vi "Supply_SetVolts.vi"(8 "error in (no error)":errorcluster, 9 "Command string":string, 10 "Volts IN [V]":dbl, 11 "KE2410 in":refnum<class "KE2410.lvclass">) -> (0 "error out":errorcluster, 2 "Compliance exceeded?":bool, 3 "KE2410 out":refnum<class "KE2410.lvclass">)   [LabVIEW 2018, in "KE2410.lvclass"]
uses:
  KE2410.lvclass
  InstrumentSetup.vi
  SupplyControl.lvclass
  InstrControl.lvclass
panel:
  out "Command sent":string
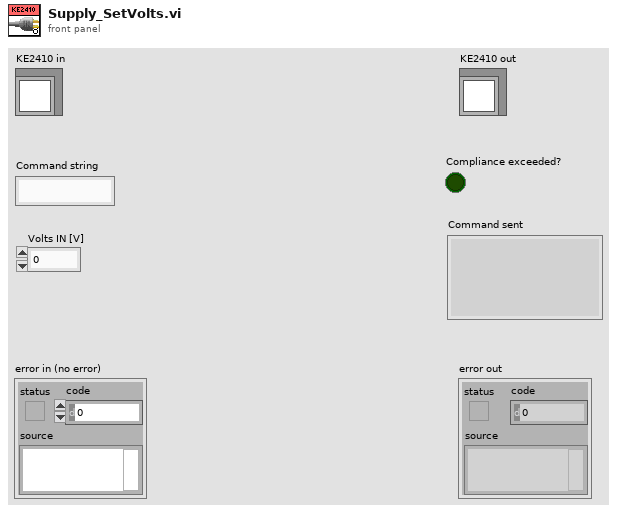
[diagram p1: front panel]
types:
  T1 = cluster{"Current Limit":sgl, "KE2410":refnum<class "KE2410.lvclass">}
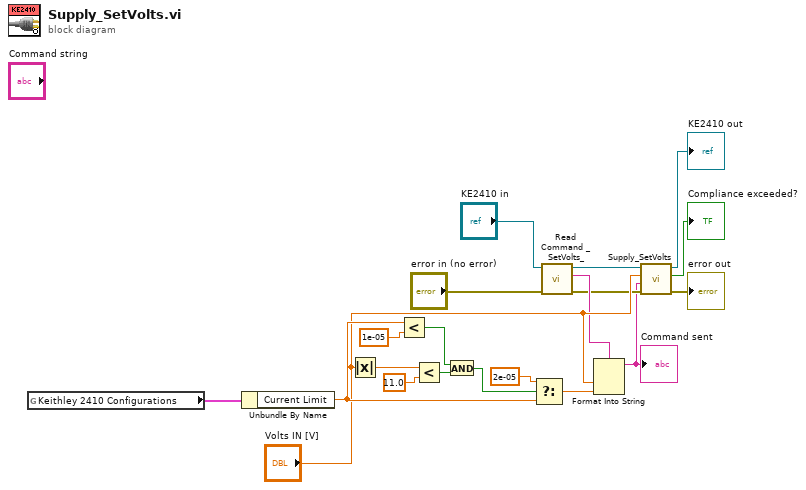
[diagram p0: block diagram]
diagram:
  n1 = global read "InstrumentSetup.vi" "Keithley 2410 Configurations"() -> (w17:T1)
  n2 = Unbundle By Name(w17) -> ("Current Limit"=w8:sgl)
  n3 = Absolute Value(x="Volts IN [V]") -> (abs(x)=w9:dbl)
  n4 = Less?(x=w8, y=1e-05) -> (x < y?=w13:bool)
  n5 = Less?(x=w9, y=11.0) -> (x < y?=w11:bool)
  n6 = And(x=w13, y=w11) -> (x .and. y?=w12:bool)
  n7 = Select(t=2e-05, s=w12, f=w8) -> (s? t:f=w16:dbl)
  n8 = call-dynamic "Read Command _SetVolts_.vi"("error in (no error)"="error in (no error)", "SupplyControl in"="KE2410 in") -> ("error out"=w3:errorcluster, "Command \"SetVolts\""=w4:string, "SupplyControl out"=w2:refnum<class "KE2410.lvclass">)  [unwired: 7 in]
  n9 = Format Into String(format string=w4, "Volts IN [V]", w16) -> (resulting string=w1:string)  [unwired: 2 in, 1 out]
  "Command sent" <- w1
  n10 = call-parent "Supply_SetVolts.vi"("error in (no error)"=w3, "Command string"=w1, "Volts IN [V]"="Volts IN [V]", "SupplyControl in"=w2) -> ("error out"=→"error out":errorcluster, "Compliance exceeded?"=→"Compliance exceeded?":bool, "SupplyControl out"=→"KE2410 out":refnum<class "KE2410.lvclass">)  [unwired: 5 in]
